vi "Internal Byte Stream Current Info.vi"(6 "error in (no error)":errorcluster, 9 "Byte Stream in":refnum<data-value>) -> (0 "error out":errorcluster, 2 "Byte Stream Size (bytes)":u64, 3 "Byte Stream":refnum<data-value>, 4 "Y Resolution":i32, 5 "X Resolution":i32)   [LabVIEW 2020]
uses:
  <vilib>/Utility/error.llb/Error Cluster From Error Code.vi
  Buffer.lvclass/Buffer.ctl
  Buffer.lvclass
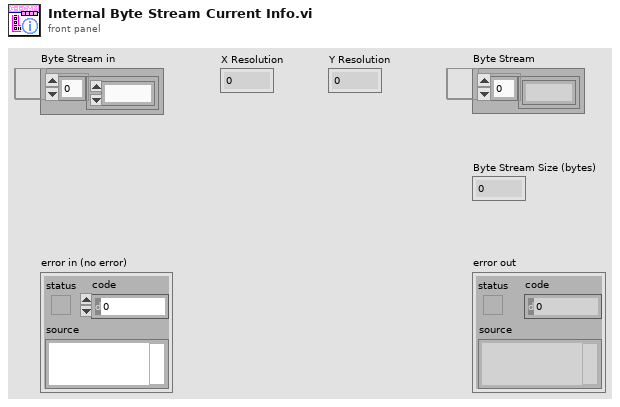
[diagram p1: front panel]
types:
  T1 = typedef "Buffer.lvclass/Image Size.ctl" = cluster{"Width":u16, "Height":u16}
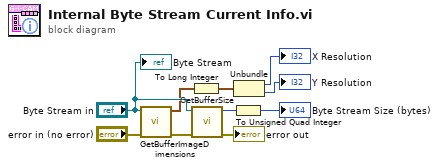
[diagram p0: block diagram]
diagram:
  n1 = call "GetBufferImageDimensions.vi"("error in (no error)"="error in (no error)", "Data Value Reference in"="Byte Stream in") -> ("error out"=w5:errorcluster, "Dims"=w4:T1)  [unwired: 8 in]
  n2 = To Long Integer(number=w4) -> (32bit integer=w3:cluster{"Width":i32, "Height":i32})
  n3 = call "GetBufferSize.vi"("error in (no error)"=w5, "Handle"="Byte Stream in") -> ("error out"=→"error out":errorcluster, "Size"=w9:i32)  [unwired: 8 in]
  n4 = To Unsigned Quad Integer(1:w9) -> (0:→"Byte Stream Size (bytes)":u64)
  n5 = Unbundle(w3) -> ("Width"=→"X Resolution":i32, "Height"=→"Y Resolution":i32)
  "Byte Stream" <- "Byte Stream in"
